vi "Shifter Control Loop.vi"(8 "error in (no error)":errorcluster) -> ()   [LabVIEW 2011]
uses:
  Shared/Shifter State.ctl
  <vilib>/Rock Robotics/WPI/Solenoid/WPI_SolenoidValue.ctl
  Robot Global Data.vi
  <vilib>/Rock Robotics/WPI/Solenoid/WPI_SolenoidSetEnum.vi
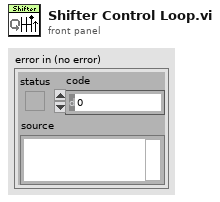
[diagram p1: front panel]
types:
  T1 = typedef "Shifter State.ctl" = enum16{"Unknown", "Low", "High"}
  T2 = typedef "WPI_SolenoidDevRef.ctl" = cluster{"DevStatus":errorcluster, "Solenoid Module":T3, "Forward Solenoid Channel":T4, "Reverse Solenoid Channel":T4}
  T3 = typedef "FPGA_TypedefSolenoidModule.ctl" = enum16{"Solenoid Module 1", "Solenoid Module 2"}
  T4 = typedef "WPI_SolenoidChannel.ctl" = enum8{"Solenoid 1", "Solenoid 2", "Solenoid 3", "Solenoid 4", "Solenoid 5", "Solenoid 6", "Solenoid 7", "Solenoid 8", "Invalid"}
  T5 = typedef "WPI_RelayDevRef.ctl" = cluster{"DevStatus":errorcluster, "Relay Channel":T6, "Digital Module":T7, "Relay Direction":T8}
  T6 = typedef "FPGA_DIORelayChannel.ctl" = enum8{"Relay 1", "Relay 2", "Relay 3", "Relay 4", "Relay 5", "Relay 6", "Relay 7", "Relay 8", "Invalid"}
  T7 = typedef "FPGA_TypedefDigitalModule.ctl" = enum16{"Digital Module 1", "Digital Module 2"}
  T8 = typedef "WPI_RelayDirection.ctl" = enum16{"Both directions", "Forward only", "Reverse only"}
  T9 = typedef "WPI_SolenoidValue.ctl" = enum16{"Off", "On", "Forward", "Reverse"}
  T10 = typedef "Drive Base Dashboard Package.ctl" = cluster{"Left":dbl, "Right":dbl, "Shifter":T1}
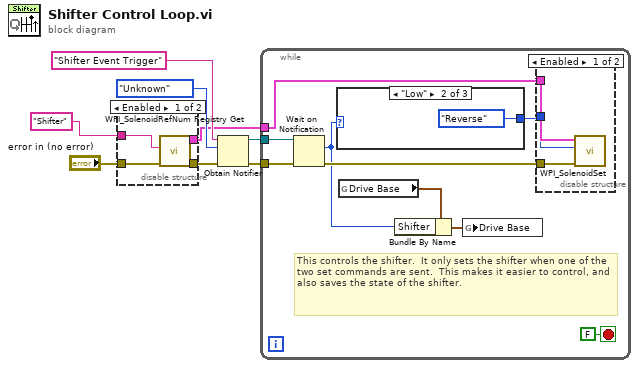
[diagram p0: block diagram]
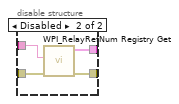
[diagram p2: hidden frame]
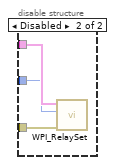
[diagram p3: hidden frame]
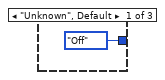
[diagram p4: hidden frame]
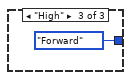
[diagram p5: hidden frame]
diagram:
  n1 = disable-structure shown="Enabled" {
    disable-tunnel: "Shifter" ("refnum name") -> [w12 w16]
    disable-tunnel: [w11 w13] -> w3
    disable-tunnel: [w10 w14] -> w2
    disable-tunnel: "error in (no error)" -> [w9 w15]
    frame Enabled {
      n2 = call <vilib>:"WPI_SolenoidRefNum Registry Get.vi"("error in (no error)"=w9, "refnum name"=w12) -> ("error out"=w10:errorcluster, "SolenoidDevRef"=w11:T2)  [unwired: 8 in]
    }
    frame Disabled {
      n3 = call <vilib>:"WPI_RelayRefNum Registry Get.vi"("error in (no error)"=w15, "refnum name"=w16) -> ("error out"=w14:errorcluster, "RelayDevRef"=w13:T5)  [unwired: 8 in]
    }
  }
  n4 = Obtain Notifier(name (unnamed)="Shifter Event Trigger", notification data type=Shifter_State."Unknown", error in (no error)=w2) -> (notifier out=w7:refnum<notifier>, error out=w6:errorcluster)  [unwired: 1 in, 1 out]
  n5 = while {
    tunnel: w7 -> [w25]
    tunnel: w6 -> [w24]
    tunnel: w3 -> [w21]
    stop <- FALSE stop-if-true
    # "This controls the shifter.  It only sets the shifter when one of the two set commands are sent.  This makes it easier to control, and also saves the state of the shifter."
    n6 = Wait on Notification(notifier=w25, error in (no error)=w24) -> (notification=w17:T1, error out=w22:errorcluster)  [unwired: 2 in, 2 out]
    n7 = case shown="\"Low\"" w17 {
      tunnel: [WPI_SolenoidValue."Off" ("t") WPI_SolenoidValue."Reverse" ("Value") WPI_SolenoidValue."Forward" ("Value")] -> w18
      frame "Unknown", Default {
      }
      frame "Low" {
      }
      frame "High" {
      }
    }
    n8 = global read "Robot Global Data.vi" "Drive Base"() -> (w20:T10)
    n9 = Bundle By Name(cluster=w20, "Shifter"=w17) -> (w19:T10)
    n10 = global write "Robot Global Data.vi" "Drive Base"(w19) -> ()
    n11 = disable-structure shown="Enabled" {
      disable-tunnel: w22 -> [w28 w30]
      disable-tunnel: w21 -> [w27 w31]
      disable-tunnel: w18 -> [w26 w29]
      frame Enabled {
        n12 = call-poly <vilib>:"WPI_SolenoidSet.vi"("error in (no error)"=w28, "Value"=w26, "SolenoidDevRef"=w27) -> ()  [unwired: 7 in, 2 out]
      }
      frame Disabled {
        n13 = call <vilib>:"WPI_RelaySet.vi"("error in (no error)"=w30, "RelayValue"=w29, "RelayDevRef"=w31) -> ()  [unwired: 7 in, 2 out]
      }
    }
  }
